vi "Invalid Iteration Error.vi"(7 "error source vi name":string, 8 "error in (no error)":errorcluster, 9 "actual iteration":u64, 10 "expected iteration":u64, 11 "Transfer Group in":refnum<class "Transfer Group.lvclass">) -> (0 "error out":errorcluster, 3 "Transfer Group out":refnum<class "Transfer Group.lvclass">)   [LabVIEW 2017, in "DSF Core.lvlib" / "Transfer Group.lvclass"]
uses:
  Transfer Group.lvclass
  Errors.ctl
  Transfer Group.lvclass/Transfer Group.ctl
  VIs/Constants/Engine Library Name.vi
  <vilib>/NI/Memory Manager/VIs/Write Numeric Scalar to Source (Base10 U64).vi
  <vilib>/NI/Memory Manager/VIs/New Error Cluster (512B).vi
  DSF Core.lvlib
  <vilib>/NI/Memory Manager/Static Errors.lvlib
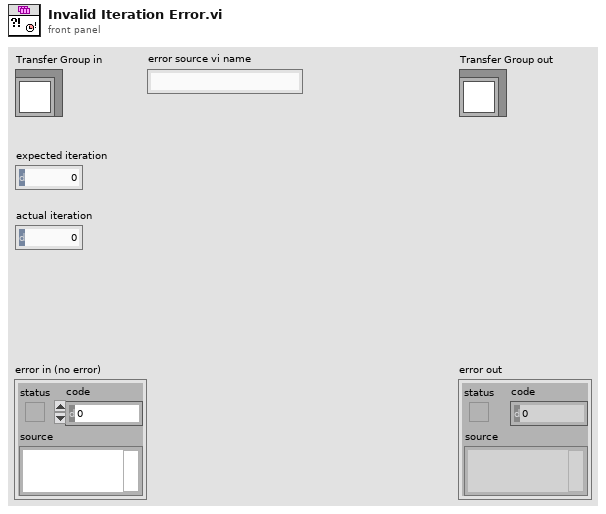
[diagram p1: front panel]
types:
  T1 = typedef "DSF Core.lvlib/Transfer Group.lvclass/Errors.ctl" = enum16{"Return Timeout", "Invalid Iteration"}
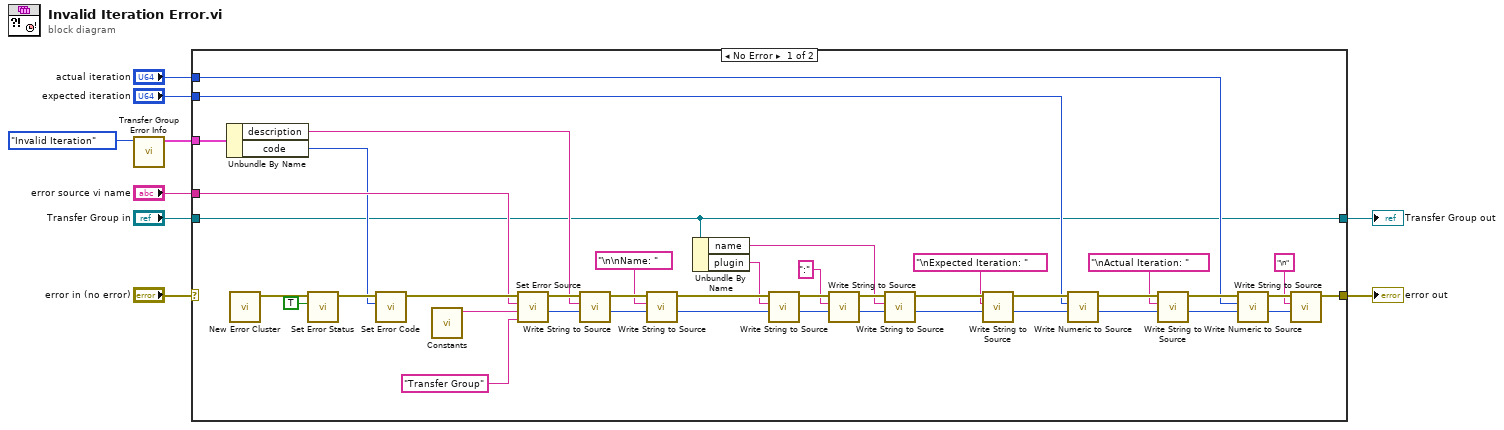
[diagram p0: block diagram]
diagram:
  n1 = call "Transfer Group Error Info.vi"("errors"=Errors."Invalid Iteration") -> ("error info"=w2:cluster{"code":i32, "description":string})  [unwired: 10 in]
  n2 = case shown="No Error" "error in (no error)" {
    selector: "error in (no error)" -> [_ w51]
    tunnel: [w38 w51] -> w8
    tunnel: [w13 w52] -> w7
    tunnel: "Transfer Group in" -> [w13 w52]
    tunnel: "error source vi name" -> [w42 _]
    tunnel: "expected iteration" -> [w27 _]
    tunnel: w2 -> [w34 _]
    tunnel: "actual iteration" -> [w26 _]
    frame No Error {
      n3 = Unbundle By Name(w34) -> ("description"=w28:string, "code"=w33:i32)
      n4 = call-poly <vilib>:"New Error Cluster.vi"() -> ("error out"=w50:errorcluster)  [unwired: 10 in, 1 out]
      n5 = call <vilib>:"Set Error Status.vi"("status (T)"=TRUE, "error in"=w50) -> ("error out"=w49:errorcluster)  [unwired: 8 in, 1 out]
      n6 = call <vilib>:"Set Error Code.vi"("code"=w33, "error in"=w49) -> ("error out"=w48:errorcluster)  [unwired: 8 in, 1 out]
      n7 = call-poly "Constants.vi"() -> ("Engine Library Name"=w47:string)  [unwired: 11 in]
      n8 = call <vilib>:"Set Error Source.vi"("class name (\"\")"="Transfer Group" ("Engine Library Name"), "library name (\"\")"=w47, "vi name"=w42, "error in"=w48) -> ("initial offset"=w31:i32, "error out"=w32:errorcluster)  [unwired: 6 in]
      n9 = call <vilib>:"Write String to Source.vi"("offset"=w31, "string"=w28, "error in"=w32) -> ("new offset"=w15:i32, "error out"=w16:errorcluster)  [unwired: 7 in]
      n10 = call <vilib>:"Write String to Source.vi"("offset"=w15, "string"="\n\nName: ", "error in"=w16) -> ("new offset"=w24:i32, "error out"=w25:errorcluster)  [unwired: 7 in]
      n11 = Unbundle By Name(w13) -> ("name"=w19:string, "plugin"=w23:string)
      n12 = call <vilib>:"Write String to Source.vi"("offset"=w24, "string"=w23, "error in"=w25) -> ("new offset"=w22:i32, "error out"=w18:errorcluster)  [unwired: 7 in]
      n13 = call <vilib>:"Write String to Source.vi"("offset"=w22, "string"=":", "error in"=w18) -> ("new offset"=w20:i32, "error out"=w21:errorcluster)  [unwired: 7 in]
      n14 = call <vilib>:"Write String to Source.vi"("offset"=w20, "string"=w19, "error in"=w21) -> ("new offset"=w11:i32, "error out"=w12:errorcluster)  [unwired: 7 in]
      n15 = call <vilib>:"Write String to Source.vi"("offset"=w11, "string"="\nExpected Iteration: ", "error in"=w12) -> ("new offset"=w45:i32, "error out"=w46:errorcluster)  [unwired: 7 in]
      n16 = call-poly <vilib>:"Write Numeric to Source.vi"("offset"=w45, "value"=w27, "error in"=w46) -> ("new offset"=w43:i32, "error out"=w44:errorcluster)  [unwired: 7 in]
      n17 = call <vilib>:"Write String to Source.vi"("offset"=w43, "string"="\nActual Iteration: ", "error in"=w44) -> ("new offset"=w40:i32, "error out"=w41:errorcluster)  [unwired: 7 in]
      n18 = call-poly <vilib>:"Write Numeric to Source.vi"("offset"=w40, "value"=w26, "error in"=w41) -> ("new offset"=w37:i32, "error out"=w39:errorcluster)  [unwired: 7 in]
      n19 = call <vilib>:"Write String to Source.vi"("offset"=w37, "string"="\n", "error in"=w39) -> ("error out"=w38:errorcluster)  [unwired: 7 in, 1 out]
    }
    frame Error {
      # "Incoming error. Pass through."
    }
  }
  "error out" <- w8
  "Transfer Group out" <- w7
